vi "Default Selector (Strings).vi"(9 "Null String":string, 10 "Default Sting":string, 11 "Input String":string) -> (3 "Output String":string)   [LabVIEW 2018]
panel:
  # "Inputs"
  # "Outputs"
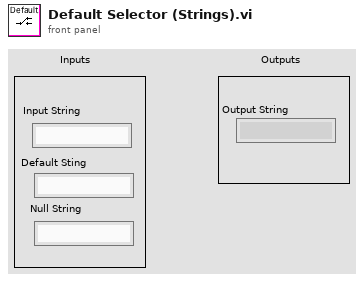
[diagram p1: front panel]
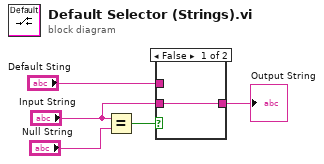
[diagram p0: block diagram]
diagram:
  n1 = Equal?(x="Input String", y="Null String") -> (x = y?=w5:bool)
  n2 = case shown="False" w5 {
    tunnel: "Input String" -> [w6 _]
    tunnel: [w6 w7] -> w1
    tunnel: "Default Sting" -> [_ w7]
    frame False {
    }
    frame True {
    }
  }
  "Output String" <- w1
